vi "Read state.vi"(8 "error in (no error)":errorcluster, 11 "MccRotTrack in":refnum<class "MccRotTrack.lvclass">) -> (0 "error out":errorcluster, 2 "MountTrackStates":T1, 3 "MccRotTrack out":refnum<class "MccRotTrack.lvclass">)   [LabVIEW 2022 SP3, in "TCSDataDefinitions.lvlib" / "TCSMountControlCommand.lvlib" / "CommandsForRotatorAxis.lvlib" / "MccRotTrack.lvclass"]
uses:
  MccRotTrack.lvclass
  Enumerations/MountTrackStates.ctl
  MccRotTrack.lvclass/MccRotTrack.ctl
  TCSMountControlCommand.lvlib
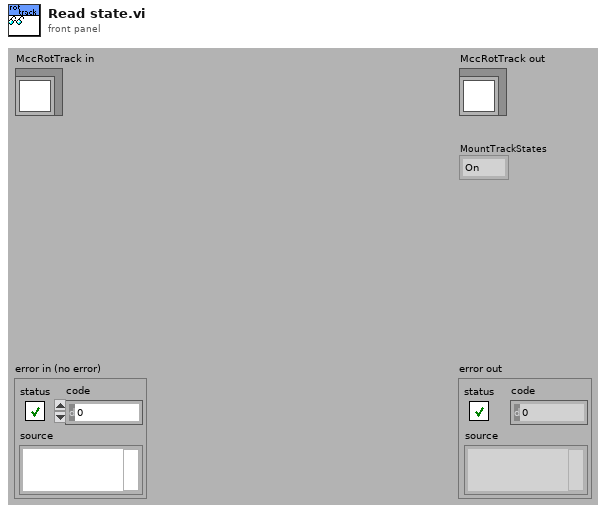
[diagram p1: front panel]
types:
  T1 = typedef "TCSDataDefinitions.lvlib/TCSMountControlCommand.lvlib/MountTrackStates.ctl" = enum16{"On", "Off"}
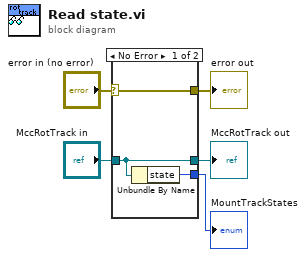
[diagram p0: block diagram]
diagram:
  n1 = case shown="No Error" "error in (no error)" {
    selector: "error in (no error)" -> [w8 w9]
    tunnel: [w8 w9] -> w4
    tunnel: [w7 w10] -> w2
    tunnel: "MccRotTrack in" -> [w7 w10]
    tunnel: [w6 _] -> w1
    frame No Error {
      n2 = Unbundle By Name(w7) -> ("state"=w6:T1)
    }
    frame Error {
    }
  }
  "error out" <- w4
  "MccRotTrack out" <- w2
  "MountTrackStates" <- w1
